vi "CD Init_Prepare Async Data_MC Tx.vi"(8 "error in (no error)":errorcluster, 10 "Card Parameters (in)":T5, 11 "Channels In":T12[](array[typedef]) {"RTs"."Mode Codes"."param item refs" format="%.0x"; "RTs"."Mode Codes"."Timestamp Channel Data Reference" format="%.0x"; "RTs"."subAddresses"."param item refs" format="%.0x"; "RTs"."subAddresses"."Timestamp Channel Data Reference" format="%.0x"; "RTs"."Status Channel Data Reference" format="%.0x"; "RTs"."Command Channels Refs" format="%.0x"; "BC"."Acyclic Frames Trigger Channels Refs" format="%.0x"; "BC"."Command Channels Refs" format="%.0x"; "BC"."messages"."Timestamp Channel Data Reference" format="%.0x"; "BC"."messages"."Status Channel Data Refs" format="%.0x"; "BC"."messages"."param item refs" format="%.0x"; "BC"."messages"."param Block Data Refs"."Data Reference" format="%.0x"}) -> (0 "error out":errorcluster, 1 "param map (MC Rx)":T1, 2 "Raw Values (RT to BC)":T7, 3 "Map (MC Tx)":T9[](array[typedef]) {"Word Data Reference" format="%.0x"})   [LabVIEW 2020, in "Ballard MIL-1553 Engine.lvlib"]
doc: "This VI creates a static association between NI-VS FIFO Channel Index and Physical Channel, Label Index, Parameter Index for Parameter Channel of a Tx Scheduled Label."
uses:
  Ballard MIL-1553 Engine.lvlib
  Shared/Controls and Global/RT Channel.ctl
  Shared/Controls and Global/RT BC.ctl
  <vilib>/NI VeriStand/Custom Device API/Custom Device Item Ref.ctl
  Shared/Controls and Global/RT Message.ctl
  Shared/Controls and Global/RT messageType.ctl
  Shared/Controls and Global/RT CWD1.ctl
  Shared/Controls and Global/RT CWD2.ctl
  <vilib>/NI VeriStand/Custom Device API/Data Reference.ctl
  <vilib>/NI VeriStand/Custom Device API/Block Data Reference.ctl
  System Explorer/SubVIs/Parse Parameters File/param_map_sysdef_type.ctl
  Azdo/emea-ni-vscd_Configurator/source/ConfiguratorConsumer/Ballard_1553/controls/param_type.ctl
  Azdo/emea-ni-vscd_Configurator/source/ConfiguratorConsumer/Ballard_1553/controls/param_signalType_type.ctl
  Azdo/emea-ni-vscd_Configurator/source/ConfiguratorConsumer/Ballard_1553/controls/param_encoding_type.ctl
  Shared/Controls and Global/RT Remote Terminal.ctl
  Shared/Controls and Global/RT Remote Terminal_rtMode.ctl
  Shared/Controls and Global/RT Remote Terminal_RT subAddress.ctl
  Shared/Controls and Global/RT Remote Terminal_RT direction.ctl
  Shared/Controls and Global/RT Remote Terminal_RT Mode Code.ctl
  Controls/RT Async_Map RT2BC.ctl
  Controls/RT Async_Map_Type.ctl
  Controls/RT Async_Raw Values.ctl
  Controls/RT Async_Raw Values to Messages Index_Association.ctl
  Controls/Card Parameters.ctl
  Shared/Controls and Global/Initialization Method.ctl
  Controls/Asynchronous - Parameter map_type.ctl
  Shared/EncodeDecode/_typedefs/parameter_config_type.ctl
  Shared/EncodeDecode/_typedefs/parameter_config_type_type.ctl
  Shared/EncodeDecode/_typedefs/parameter_config_encoding_type.ctl
  Controls/RT Async_Raw Values_Association.ctl
  <instrlib>/BTI1553Lib/Public/Controls/1553 RT Transfer Type.ctl
  <instrlib>/BTI1553Lib/Public/Controls/1553 Transfer Direction.ctl
  <instrlib>/BTI1553Lib/Private/RT/Configure/Get RT Xfer Handle.vi
  <vilib>/NI VeriStand/Custom Device API/Custom Device API.lvlib
  <instrlib>/BTI1553Lib/BTI1553LV.lvlib
  Shared/Ballard 1553 Shared.lvlib
  Azdo/emea-ni-vscd_Configurator/source/ConfiguratorConsumer/Ballard_1553/Ballard_1553.lvclass
  System Explorer/Ballard 1553 System Explorer.lvlib
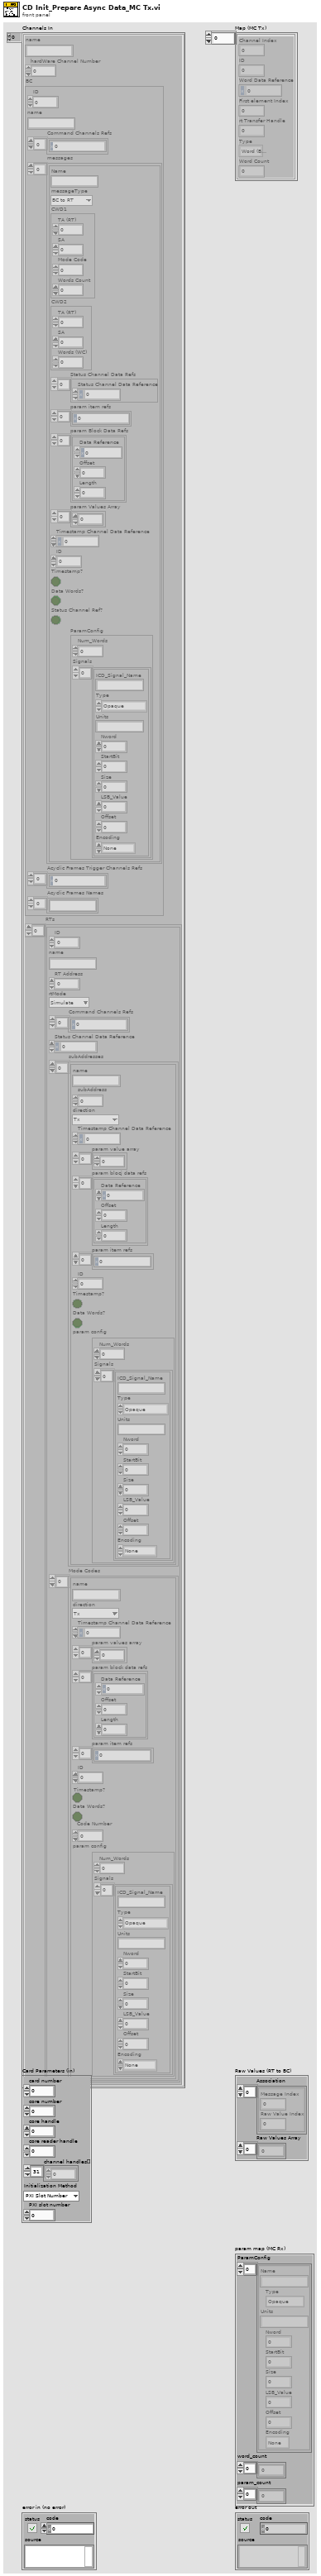
[diagram p1: front panel]
types:
  T1 = typedef "Ballard MIL-1553 Engine.lvlib/Asynchronous - Parameter map_type.ctl" = cluster{"ParamConfig":T2[], "word_count":u8[], "param_count":u8[]}
  T2 = typedef "parameter_config_type.ctl" = cluster{"Name":string, "Type":T3, "Units":string, "Nword":i32, "StartBit":i32, "Size":i32, "LSB_Value":dbl, "Offset":i32, "Encoding":T4}
  T3 = typedef "parameter_config_type_type.ctl" = enum16{"Opaque", "Enum", "Float", "Integer", "Bcd", "Bool"}
  T4 = typedef "parameter_config_encoding_type.ctl" = enum16{"None", "2-complement", "Unsigned"}
  T5 = typedef "Ballard MIL-1553 Engine.lvlib/Card Parameters.ctl" = cluster{"card number":i32, "core number":i32, "core handle":u64, "core reader handle":u64, "channel handles[]":u64[], "Initialization Method":T6, "PXI slot number":i32}
  T6 = typedef "Ballard 1553 Shared.lvlib/Initialization Method.ctl" = enum16{"PXI Slot Number", "Card Number"}
  T7 = typedef "Ballard MIL-1553 Engine.lvlib/RT Async_Raw Values.ctl" = cluster{"Association":T8[], "Raw Values Array":u16[]}
  T8 = typedef "Ballard MIL-1553 Engine.lvlib/RT Async_Raw Values to Messages Index_Association.ctl" = cluster{"Message Index":i32, "Raw Value Index":i32}
  T9 = typedef "Ballard MIL-1553 Engine.lvlib/RT Async_Map RT2BC.ctl" = cluster{"Channel Index":i32, "ID":i32, "Word Data Reference":T10, "First element Index":i32, "rt Transfer Handle":u64, "Type":T11, "Word Count":i32}
  T10 = typedef "Custom Device API.lvlib/Data Reference.ctl" = i32
  T11 = typedef "Ballard MIL-1553 Engine.lvlib/RT Async_Map_Type.ctl" = enum16{"Word (BC to RT)", "Word (MC (Rx))", "Acyclic Message Trigger", "Word (RT to ..)", "Word (RT to RT)", "Word (MC (Tx))", "RT Status", "BC Commands", "RT Commands"}
  T12 = typedef "Ballard 1553 Shared.lvlib/RT Channel.ctl" = cluster{"name":string, "hardWare Channel Number":u16, "BC":T13, "RTs":T24[]}
  T13 = typedef "Ballard 1553 Shared.lvlib/RT BC.ctl" = cluster{"ID":i32, "name":string, "Command Channels Refs":T14[], "messages":T15[], "Acyclic Frames Trigger Channels Refs":T14[], "Acyclic Frames Names":string[]}
  T14 = typedef "Custom Device API.lvlib/Custom Device Item Ref.ctl" = u64
  T15 = typedef "Ballard 1553 Shared.lvlib/RT Message.ctl" = cluster{"Name":string, "messageType":T16, "CWD1":T17, "CWD2":T18, "Status Channel Data Refs":T10[], "param item refs":T14[], "param Block Data Refs":T19[], "param Values Array":u16[], "Timestamp Channel Data Reference":T10, "ID":i32, "Timestamp?":bool, "Data Words?":bool, "Status Channel Ref?":bool, "ParamConfig":T20}
  T16 = typedef "Ballard 1553 Shared.lvlib/RT messageType.ctl" = enum16{"BC to RT", "RT to BC", "RT to RT", "MC (Rx)", "MC (Tx)"}
  T17 = typedef "Ballard 1553 Shared.lvlib/RT CWD1.ctl" = cluster{"TA (RT)":i8, "SA":i8, "Mode Code":i8, "Words Count":i8}
  T18 = typedef "Ballard 1553 Shared.lvlib/RT CWD2.ctl" = cluster{"TA (RT)":i8, "SA":i8, "Words (WC)":i8}
  T19 = typedef "Custom Device API.lvlib/Block Data Reference.ctl" = cluster{"Data Reference":T10, "Offset":u64, "Length":u64}
  T20 = typedef "Ballard 1553 System Explorer.lvlib/param_map_sysdef_type.ctl" = cluster{"Num_Words":u8, "Signals":T21[]}
  T21 = typedef "ConfigurationManager.lvlib/Ballard_1553.lvclass/param_type.ctl" = cluster{"ICD_Signal_Name":string, "Type":T22, "Units":string, "Nword":i32, "StartBit":i32, "Size":i32, "LSB_Value":dbl, "Offset":i32, "Encoding":T23}
  T22 = typedef "ConfigurationManager.lvlib/Ballard_1553.lvclass/param_signalType_type.ctl" = enum16{"Opaque", "Enum", "Float", "Integer", "Bcd", "Bool"}
  T23 = typedef "ConfigurationManager.lvlib/Ballard_1553.lvclass/param_encoding_type.ctl" = enum16{"None", "2-complement", "Unsigned"}
  T24 = typedef "Ballard 1553 Shared.lvlib/RT Remote Terminal.ctl" = cluster{"ID":i32, "name":string, "RT Address":i32, "rtMode":T25, "Command Channels Refs":T14[], "Status Channel Data Reference":T10, "subAddresses":T26[], "Mode Codes":T28[]}
  T25 = typedef "Ballard 1553 Shared.lvlib/RT Remote Terminal_rtMode.ctl" = enum16{"Simulate", "Monitor", "Disable"}
  T26 = typedef "Ballard 1553 Shared.lvlib/RT Remote Terminal_RT subAddress.ctl" = cluster{"name":string, "subAddress":i8, "direction":T27, "Timestamp Channel Data Reference":T10, "param value array":u16[], "param blocj data refs":T19[], "param item refs":T14[], "ID":i32, "Timestamp?":bool, "Data Words?":bool, "param config":T20}
  T27 = typedef "Ballard 1553 Shared.lvlib/RT Remote Terminal_RT direction.ctl" = enum16{"Tx", "Rx"}
  T28 = typedef "Ballard 1553 Shared.lvlib/RT Remote Terminal_RT Mode Code.ctl" = cluster{"name":string, "direction":T27, "Timestamp Channel Data Reference":T10, "param values array":u16[], "param block data refs":T19[], "param item refs":T14[], "ID":i32, "Timestamp?":bool, "Data Words?":bool, "Code Number":i32, "param config":T20}
  T29 = typedef "Ballard MIL-1553 Engine.lvlib/RT Async_Raw Values_Association.ctl" = cluster{"Channel Data Reference":T10, "Raw Value Index":i32}
  T30 = typedef "BTI1553LV.lvlib/1553 Transfer Direction.ctl" = u32
  T31 = typedef "BTI1553LV.lvlib/1553 RT Transfer Type.ctl" = u32
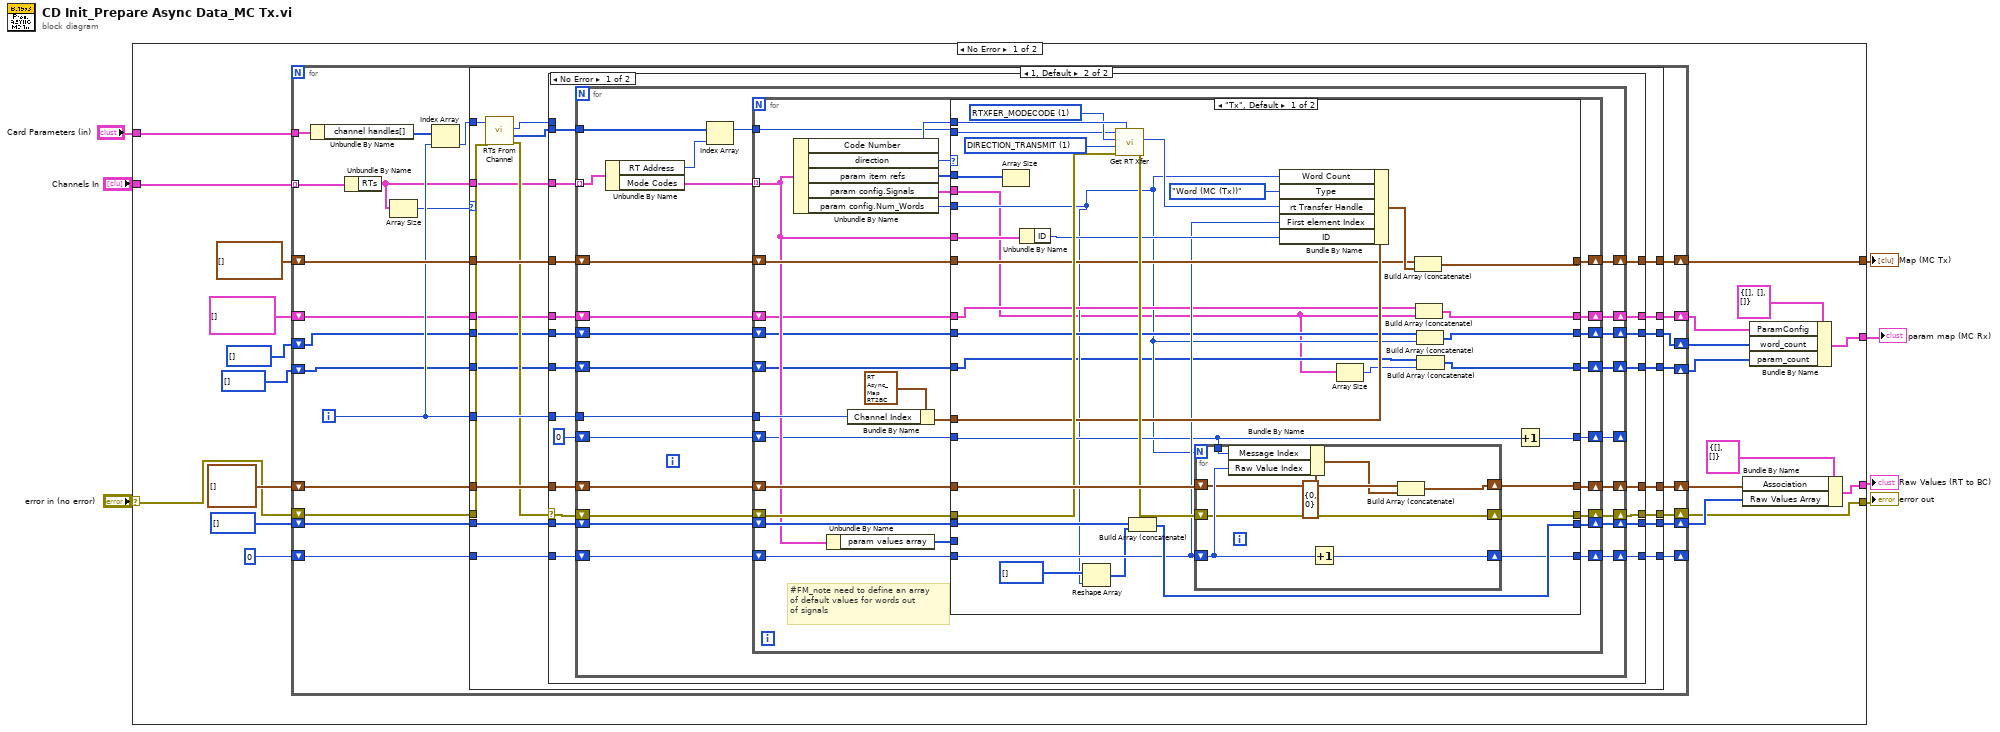
[diagram p0: block diagram]
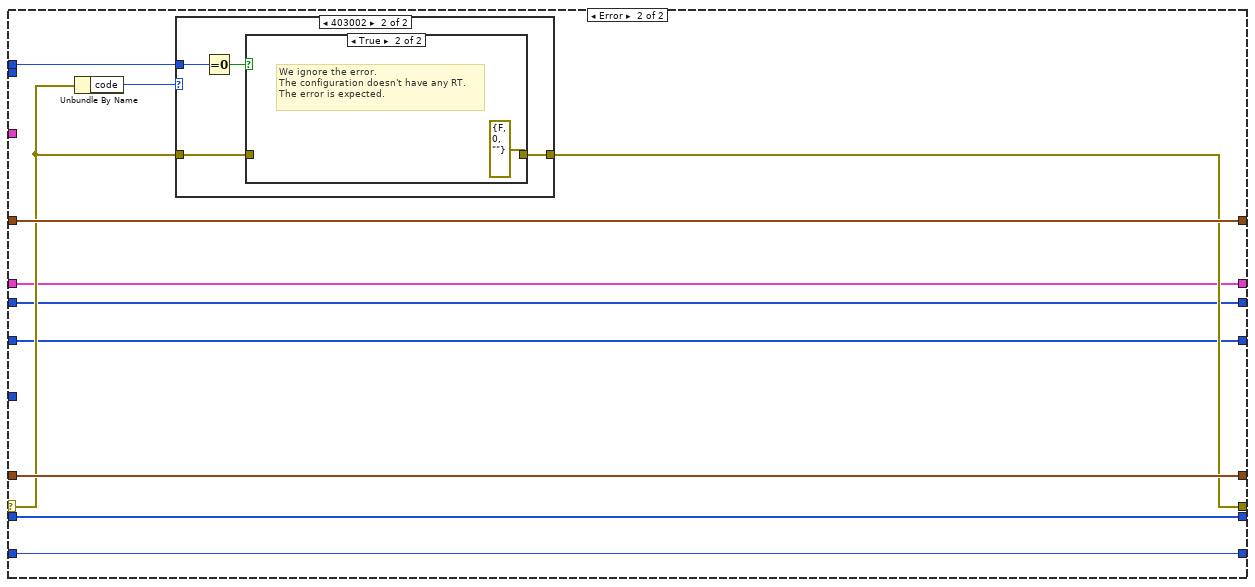
[diagram p4: hidden frame]
diagram:
  n1 = case shown="No Error" "error in (no error)" {
    selector: "error in (no error)" -> [w17 w225]
    tunnel: [w16 w225] -> w6
    tunnel: "Channels In" -> [w28 _]
    tunnel: [w26 _] -> w4
    tunnel: [w22 _] -> w3
    tunnel: "Card Parameters (in)" -> [w18 _]
    tunnel: [w14 _] -> w1
    frame No Error {
      n2 = for {
        tunnel: w28 -> [w51] mode=indexing
        shift-right: [w49] -> w26
        shift-left: T9[] [] -> [w50]
        shift-right: [w47] -> w23
        shift-left: T29[] [] -> [w48]
        shift-right: [w43] -> w20
        shift-left: u16[] [] -> [w46]
        shift-right: [w44] -> _
        shift-left: 0 -> [w45]
        tunnel: w18 -> [w42]
        shift-right: [w39] -> w16
        shift-left: w17 -> [w37]
        shift-right: [w32] -> w10
        shift-left: T2[] [] ("ParamConfig") -> [w34]
        shift-right: [w31] -> w11
        shift-left: u8[] [] ("word_count") -> [w33]
        shift-right: [w29] -> w8
        shift-left: u8[] [] ("word_count") -> [w30]
        i -> [w40]
        n3 = Unbundle By Name(w42) -> ("channel handles[]"=w41:u64[])
        n4 = Unbundle By Name(w51) -> ("RTs"=w36:T24[])
        n5 = Array Size(array=w36) -> (size(s)=w35:i32)
        n6 = Index Array(array=w41, index=w40) -> (element=w38:u64)
        n7 = case shown="1, Default" w35 {
          tunnel: w50 -> [w59 w81]
          tunnel: [w59 w80] -> w49
          tunnel: w48 -> [w58 w79]
          tunnel: [w58 w78] -> w47
          tunnel: w46 -> [w56 w77]
          tunnel: w45 -> [w55 w76]
          tunnel: [w55 w75] -> w44
          tunnel: [w56 w74] -> w43
          tunnel: w40 -> [_ w73]
          tunnel: [w57 w72] -> w39
          tunnel: w38 -> [_ w71]
          tunnel: w37 -> [w57 w70]
          tunnel: w36 -> [_ w66]
          tunnel: w34 -> [w54 w65]
          tunnel: w33 -> [w53 w64]
          tunnel: [w54 w63] -> w32
          tunnel: [w53 w62] -> w31
          tunnel: w30 -> [w52 w61]
          tunnel: [w52 w60] -> w29
          frame 0 {
          }
          frame 1, Default {
            n8 = call <instrlib>:"RTs From Channel.vi"("error in (no error)"=w70, "channel handle in"=w71) -> ("error out"=w68:errorcluster, "remote terminal handles out"=w69:u64[], "remote terminal count out"=w67:i32)  [unwired: 6 in, 1 out]
            n9 = case shown="No Error" w68 {
              selector: w68 -> [w88 w212]
              tunnel: w66 -> [w101 _]
              tunnel: w81 -> [w100 w214]
              tunnel: [w99 w214] -> w80
              tunnel: w79 -> [w98 w215]
              tunnel: [w97 w215] -> w78
              tunnel: w77 -> [w96 w216]
              tunnel: w76 -> [w95 w217]
              tunnel: [w94 w217] -> w75
              tunnel: [w93 w216] -> w74
              tunnel: w73 -> [w92 _]
              tunnel: [w91 w210] -> w72
              tunnel: w69 -> [w90 _]
              tunnel: w67 -> [_ w211]
              tunnel: w65 -> [w87 w209]
              tunnel: w64 -> [w86 w208]
              tunnel: [w85 w209] -> w63
              tunnel: [w84 w208] -> w62
              tunnel: w61 -> [w83 w207]
              tunnel: [w82 w207] -> w60
              frame No Error {
                n10 = for {
                  tunnel: w101 -> [w112] mode=indexing
                  shift-right: [w123] -> w99
                  shift-left: w100 -> [w124]
                  tunnel: w92 -> [w125]
                  shift-right: [w122] -> w97
                  shift-left: w98 -> [w118]
                  shift-right: [w121] -> w93
                  shift-left: w96 -> [w117]
                  shift-right: [w120] -> w94
                  shift-left: w95 -> [w119]
                  tunnel: w90 -> [w116]
                  shift-right: [w114] -> w91
                  shift-left: w88 -> [w115]
                  shift-right: [w108] -> _
                  shift-left: 0 -> [w109]
                  shift-right: [w105] -> w85
                  shift-left: w87 -> [w107]
                  shift-right: [w104] -> w84
                  shift-left: w86 -> [w106]
                  shift-right: [w102] -> w82
                  shift-left: w83 -> [w103]
                  n11 = Unbundle By Name(w112) -> ("RT Address"=w110:i32, "Mode Codes"=w113:T28[])
                  n12 = Index Array(array=w116, index=w110) -> (element=w111:u64)
                  n13 = for {
                    tunnel: w125 -> [w154]
                    tunnel: w113 -> [w137] mode=indexing
                    tunnel: w111 -> [w139]
                    shift-right: [w147] -> w120
                    shift-left: w119 -> [w146]
                    shift-right: [w141] -> w114
                    shift-left: w115 -> [w142]
                    shift-right: [w152] -> w123
                    shift-left: w124 -> [w153]
                    shift-right: [w149] -> w122
                    shift-left: w118 -> [w145]
                    shift-right: [w148] -> w121
                    shift-left: w117 -> [w144]
                    shift-right: [w134] -> w108
                    shift-left: w109 -> [w135]
                    shift-right: [w128] -> w104
                    shift-left: w106 -> [w132]
                    shift-right: [w131] -> w105
                    shift-left: w107 -> [w133]
                    shift-right: [w126] -> w102
                    shift-left: w103 -> [w127]
                    # "#FM_note need to define an array\nof default values for words out \nof signals"
                    n14 = Unbundle By Name(w137) -> ("Code Number"=w140:i32, "direction"=w136:T27, "param item refs"=w150:T14[], "param config.Signals"=w130:T21[], "param config.Num_Words"=w129:u8)
                    n15 = Unbundle By Name(w137) -> ("param values array"=w143:u16[])
                    n16 = Bundle By Name(cluster=T9 {"Channel Index"=0, "ID"=0, "Word Data Reference"=0, "First element Index"=0, "rt Transfer Handle"=0, "Type"=enum."Word (BC to RT)", "Word Count"=0} ("Association"), "Channel Index"=w154) -> (w151:T9)
                    n17 = case shown="\"Tx\", Default" w136 {
                      tunnel: w153 -> [w171 w206]
                      tunnel: [w170 w206] -> w152
                      tunnel: w151 -> [w176 _]
                      tunnel: w150 -> [w168 _]
                      tunnel: [w177 w205] -> w149
                      tunnel: [w189 w203] -> w148
                      tunnel: [w188 w202] -> w147
                      tunnel: w146 -> [w167 w202]
                      tunnel: w145 -> [w187 w205]
                      tunnel: w144 -> [w186 w203]
                      tunnel: w143 -> [_ _]
                      tunnel: w142 -> [w185 w204]
                      tunnel: [w183 w204] -> w141
                      tunnel: w140 -> [w182 _]
                      tunnel: w139 -> [w180 _]
                      tunnel: w137 -> [w179 _]
                      tunnel: w135 -> [w166 w201]
                      tunnel: [w169 w201] -> w134
                      tunnel: w133 -> [w165 w200]
                      tunnel: w132 -> [w163 w199]
                      tunnel: [w164 w200] -> w131
                      tunnel: w130 -> [w157 _]
                      tunnel: w129 -> [w160 _]
                      tunnel: [w162 w199] -> w128
                      tunnel: w127 -> [w158 w198]
                      tunnel: [w155 w198] -> w126
                      frame "Tx", Default {
                        w178 = T30 1 items=["DIRECTION_RECEIVE", "DIRECTION_TRANSMIT"] ("transfer direction")
                        w181 = T31 1 items=["RTXFER_SUBADDRESS", "RTXFER_MODECODE"] ("transfer type")
                        n18 = Array Size(array=w168) -> ()  [unwired: 1 out]
                        n19 = Unbundle By Name(w179) -> ("ID"=w173:i32)
                        n20 = Reshape Array(u16[] [] ("param value array"), w160) -> (w159:u16[])
                        n21 = call-poly <instrlib>:"Get RT Xfer.vi"("transfer sa number or mc number"=w182, "error in (no error)"=w185, "transfer direction"=w178, "transfer type"=w181, "remote terminal handle in"=w180) -> ("error out"=w184:errorcluster, "rt transfer handle out"=w174:u64)  [unwired: 4 in, 1 out]
                        n22 = Build Array (concatenate)(w186, w159) -> (w189:u16[])
                        n23 = for {
                          N: w160 -> [_]
                          shift-right: [w197] -> w188
                          shift-left: w167 -> [w196]
                          shift-right: [w194] -> w183
                          shift-left: w184 -> [w194]
                          shift-right: [w191] -> w177
                          shift-left: w187 -> [w195]
                          tunnel: w166 -> [w190]
                          n24 = Bundle By Name(cluster=T8 {"Message Index"=0, "Raw Value Index"=0}, "Message Index"=w190, "Raw Value Index"=w196) -> (w192:T8)
                          n25 = Increment(x=w196) -> (x+1=w197:i32)
                          n26 = Build Array (concatenate)(w195, w192) -> (w191:T29[])
                        }
                        n27 = Bundle By Name(cluster=w176, "Word Count"=w160, "Type"=RT_Async_Map_Type."Word (MC (Tx))", "rt Transfer Handle"=w174, "First element Index"=w167, "ID"=w173) -> (w172:T9)
                        n28 = Array Size(array=w157) -> (size(s)=w156:i32)
                        n29 = Build Array (concatenate)(w171, w172) -> (w170:T9[])
                        n30 = Build Array (concatenate)(w165, w157) -> (w164:T21[])
                        n31 = Build Array (concatenate)(w163, w160) -> (w162:u8[])
                        n32 = Build Array (concatenate)(w158, w156) -> (w155:i32[])
                        n33 = Increment(x=w166) -> (x+1=w169:i32)
                      }
                      frame "Rx" {
                      }
                    }
                  }
                }
              }
              frame Error {
                n34 = Unbundle By Name(w212) -> ("code"=w213:i32)
                n35 = case shown="403002" w213 {
                  tunnel: w212 -> [w218 w220]
                  tunnel: w211 -> [_ w222]
                  tunnel: [w218 w219] -> w210
                  frame 0, Default {
                  }
                  frame 403002 {
                    n36 = Equal To 0?(x=w222) -> (x = 0?=w221:bool)
                    n37 = case shown="True" w221 {
                      tunnel: w220 -> [w223 _]
                      tunnel: [w223 errorcluster {"status"=FALSE, "code"=0, "source"=""} ("error IO")] -> w219
                      frame False {
                      }
                      frame True {
                        # "We ignore the error.\nThe configuration doesn't have any RT.\nThe error is expected."
                      }
                    }
                  }
                }
              }
            }
          }
        }
      }
      n38 = Bundle By Name(cluster=T7 {"Association"=[], "Raw Values Array"=[]} ("Raw Values"), "Association"=w23, "Raw Values Array"=w20) -> (w22:T7)
      n39 = Bundle By Name(cluster=T1 {"ParamConfig"=[], "word_count"=[], "param_count"=[]}, "ParamConfig"=w10, "word_count"=w11, "param_count"=w8) -> (w14:T1)
    }
    frame Error {
    }
  }
  "error out" <- w6
  "Map (MC Tx)" <- w4
  "Raw Values (RT to BC)" <- w3
  "param map (MC Rx)" <- w1
